vi "CalculateSpecificationBuildOrder.vi"(6 "UpdateList":T1, 8 "error in (no error)":errorcluster, 11 "SolutionBuilder in":refnum<class "SolutionBuilder.lvclass">) -> (0 "error out":errorcluster, 3 "SolutionBuilder out":refnum<class "SolutionBuilder.lvclass">)   [LabVIEW 2020, in "SolutionBuilder.lvlib" / "SolutionBuilder.lvclass"]
uses:
  SolutionBuilder.lvclass
  EventUpdateList.ctl
  SolutionBuilder.lvclass/SolutionBuilder.ctl
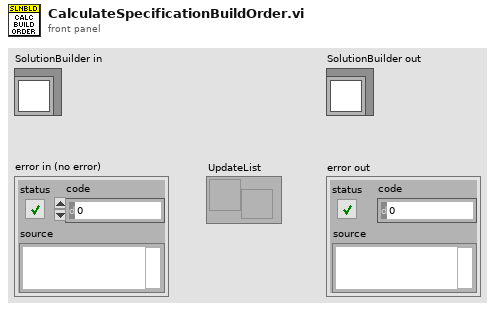
[diagram p1: front panel]
types:
  T1 = typedef "SolutionBuilder.lvlib/SolutionBuilder.lvclass/EventUpdateList.ctl" = refnum<user-event>
  T2 = typedef "SolutionBuilder.lvlib/SolutionBuilder.lvclass/ItemInfo.ctl" = map{string, T3}
  T3 = typedef "SolutionBuilder.lvlib/SolutionBuilder.lvclass/ProjectInfo.ctl" = cluster{"Deps":set{string}, "FileInfo":T4}
  T4 = typedef "SolutionBuilder.lvlib/SolutionBuilder.lvclass/FileInfo.ctl" = cluster{"Library ref":refnum<vi>, "Target path":path, "Source name":string, "Build spec name":string}
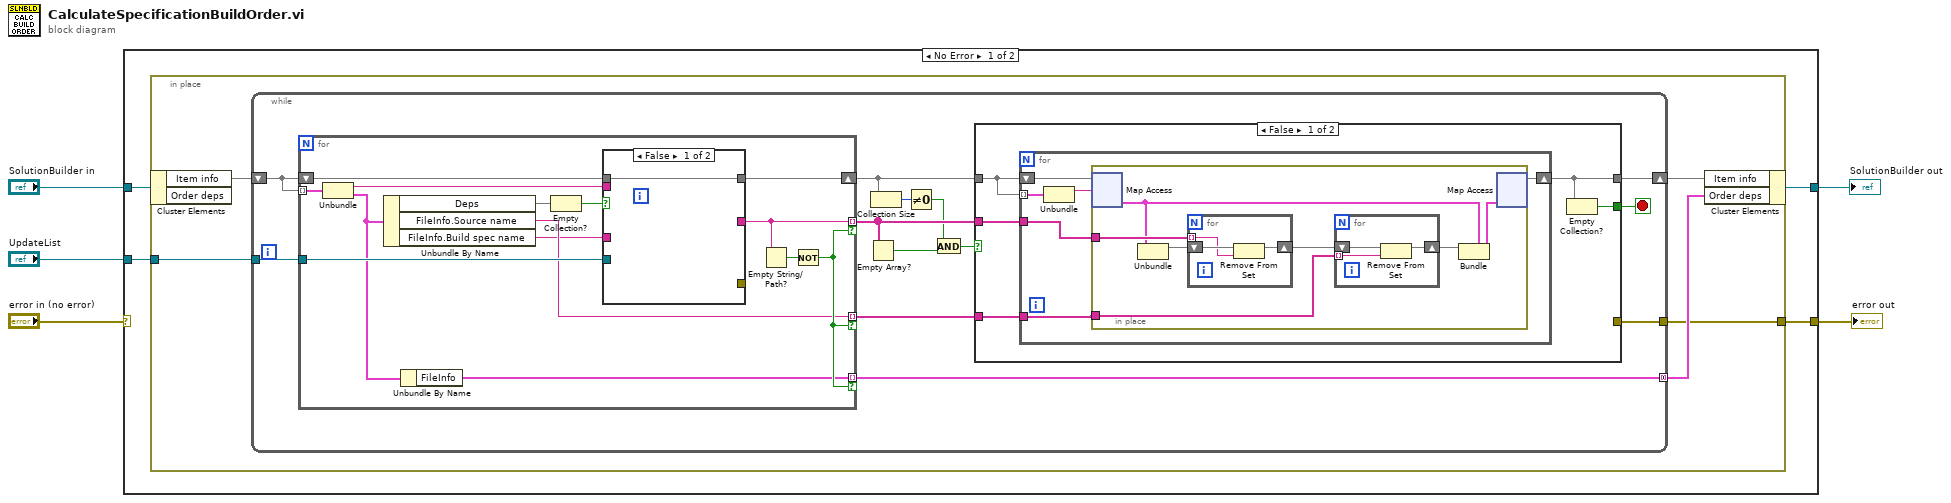
[diagram p0: block diagram]
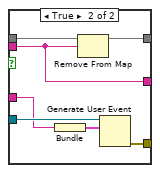
[diagram p2: hidden frame]
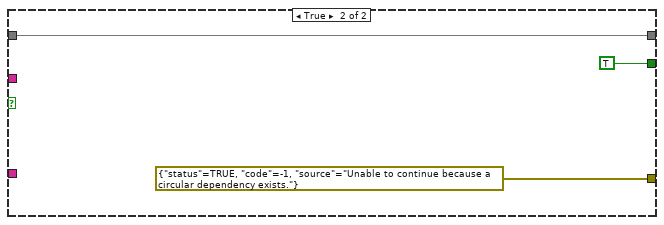
[diagram p3: hidden frame]
diagram:
  n1 = case shown="No Error" "error in (no error)" {
    selector: "error in (no error)" -> [_ w78]
    tunnel: "UpdateList" -> [w9 _]
    tunnel: "SolutionBuilder in" -> [w8 w77]
    tunnel: [w7 w77] -> w3
    tunnel: [w6 w78] -> w1
    frame No Error {
      n2 = in-place {
        in-place-border: w9 -> [w14]
        in-place-border: [w10] -> w6
        n3 = in-place-cluster #1(w8) -> ("Item info"=w13:T2)  [unwired: 1 out]
        n4 = while {
          shift-right: [w24] -> w12
          shift-left: w13 -> [w27]
          tunnel: [w25] -> w11 mode=concatenating
          tunnel: w14 -> [w23]
          tunnel: [w15] -> w10
          stop <- w26 stop-if-true
          n5 = for {
            tunnel: w27 -> [w41] mode=indexing
            shift-right: [w39] -> w21
            shift-left: w27 -> [w40]
            tunnel: [w31] -> w25 mode=indexing if=w35
            tunnel: [w29] -> w20 mode=indexing if=w35
            tunnel: w23 -> [w37]
            tunnel: [w33] -> w22 mode=indexing if=w35
            n6 = Unbundle(w41) -> ("Targetfile name"=w36:string, "ProjectInfo"=w32:T3)
            n7 = Unbundle By Name(w32) -> ("Deps"=w34:set{string}, "FileInfo.Source name"=w33:string, "FileInfo.Build spec name"=w30:string)
            n8 = Unbundle By Name(w32) -> ("FileInfo"=w31:T4)
            n9 = Empty Collection?(1:w34) -> (0:w28:bool)
            n10 = case shown="False" w28 {
              tunnel: w40 -> [w42 w49]
              tunnel: [w42 w48] -> w39
              tunnel: w37 -> [_ w47]
              tunnel: w36 -> [_ w44]
              tunnel: w30 -> [_ w46]
              tunnel: [_ w44] -> w29
              tunnel: [_ w43] -> _
              frame False {
              }
              frame True {
                n11 = Bundle("Build spec name"=w46) -> (w45:cluster{"Build spec name":string})  [unwired: 1 in]
                n12 = Remove From Map(10:w44, 11:w49) -> (3:w48:T2)  [unwired: 2 out]
                n13 = Generate User Event(user event=w47, event data cluster=w45) -> (error out=w43:errorcluster)  [unwired: 2 in, 1 out]
              }
            }
            n14 = Empty String/Path?(string/path=w29) -> (empty?=w38:bool)
            n15 = Not(x=w38) -> (.not. x?=w35:bool)
          }
          n16 = Empty Array?(array=w20) -> (empty?=w18:bool)
          n17 = Collection Size(1:w21) -> (0:w19:i32)
          n18 = Not Equal To 0?(x=w19) -> (x != 0?=w17:bool)
          n19 = And(x=w17, y=w18) -> (x .and. y?=w16:bool)
          n20 = case shown="False" w16 {
            tunnel: [w54 TRUE ("empty?")] -> w26
            tunnel: w21 -> [w53 w76]
            tunnel: w20 -> [w52 _]
            tunnel: [w51 w76] -> w24
            tunnel: w22 -> [w50 _]
            tunnel: [_ errorcluster {"status"=TRUE, "code"=-1, "source"="Unable to continue because a circular dependency exists."} ("error IO")] -> w15
            frame False {
              n21 = for {
                shift-right: [w56] -> w51
                shift-left: w53 -> [w59]
                tunnel: w53 -> [w60] mode=indexing
                tunnel: w52 -> [w57]
                tunnel: w50 -> [w55]
                n22 = Unbundle(w60) -> ("Targetfile name"=w58:string)  [unwired: 1 out]
                n23 = in-place {
                  in-place-border: w57 -> [w66]
                  in-place-border: w55 -> [w61]
                  n24 = in-place-map #2(w59, w58) -> (w65:T3)  [unwired: 1 in, 1 out]
                  n25 = Unbundle(w65) -> ("Deps"=w67:set{string})  [unwired: 1 out]
                  n26 = for {
                    tunnel: w66 -> [w72] mode=indexing
                    shift-right: [w71] -> w63
                    shift-left: w67 -> [w73]
                    n27 = Remove From Set(10:w72, 11:w73) -> (3:w71:set{string})  [unwired: 1 out]
                  }
                  n28 = for {
                    tunnel: w61 -> [w69] mode=indexing
                    shift-right: [w68] -> w62
                    shift-left: w63 -> [w70]
                    n29 = Remove From Set(10:w69, 11:w70) -> (3:w68:set{string})  [unwired: 1 out]
                  }
                  n30 = Bundle(cluster=w65, "Deps"=w62) -> (w64:T3)  [unwired: 1 in]
                  n31 = in-place-map #2(w64) -> (w56:T2)  [unwired: 1 in, 2 out]
                }
              }
              n32 = Empty Collection?(1:w51) -> (0:w54:bool)
            }
            frame True {
            }
          }
        }
        n33 = in-place-cluster #1("Item info"=w12, "Order deps"=w11) -> (w7:refnum<class "SolutionBuilder.lvclass">)
      }
    }
    frame Error {
    }
  }
  "error out" <- w1
  "SolutionBuilder out" <- w3
